vi "PCO_RecorderGetSettings.vi"(0 "phRec":u64, 5 "phCam":u64, 11 "error in (no error)":errorcluster {"code" format="%x"}) -> (2 "wHeight":u16, 3 "dwReqImgCount":u32, 4 "phRec out":u64, 6 "ErrorMessage":i32 format="%x", 8 "dwRecMode":u32, 10 "dwMaxImgCount":u32, 13 "wMetadataLines":u16, 14 "wWidth":u16, 15 "error out":errorcluster {"code" format="%x"})   [LabVIEW 2019, in "Recorder.lvlib"]
doc: "<b>Description:</b>\nThis function retrieves the current recorder settings for a specific camera.\n\n<b>Supported camera type:</b>\nAll cameras"
uses:
  Recorder.lvlib
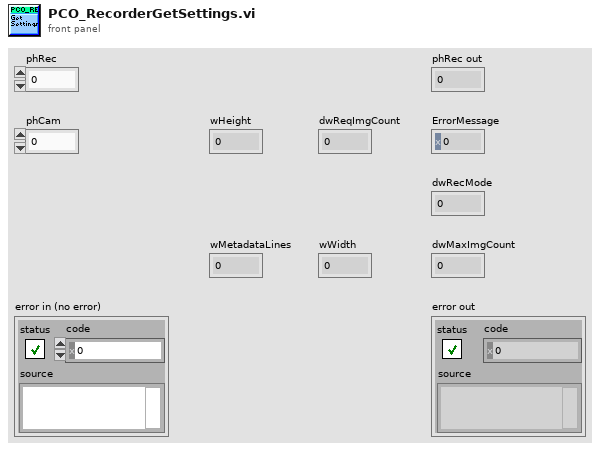
[diagram p1: front panel]
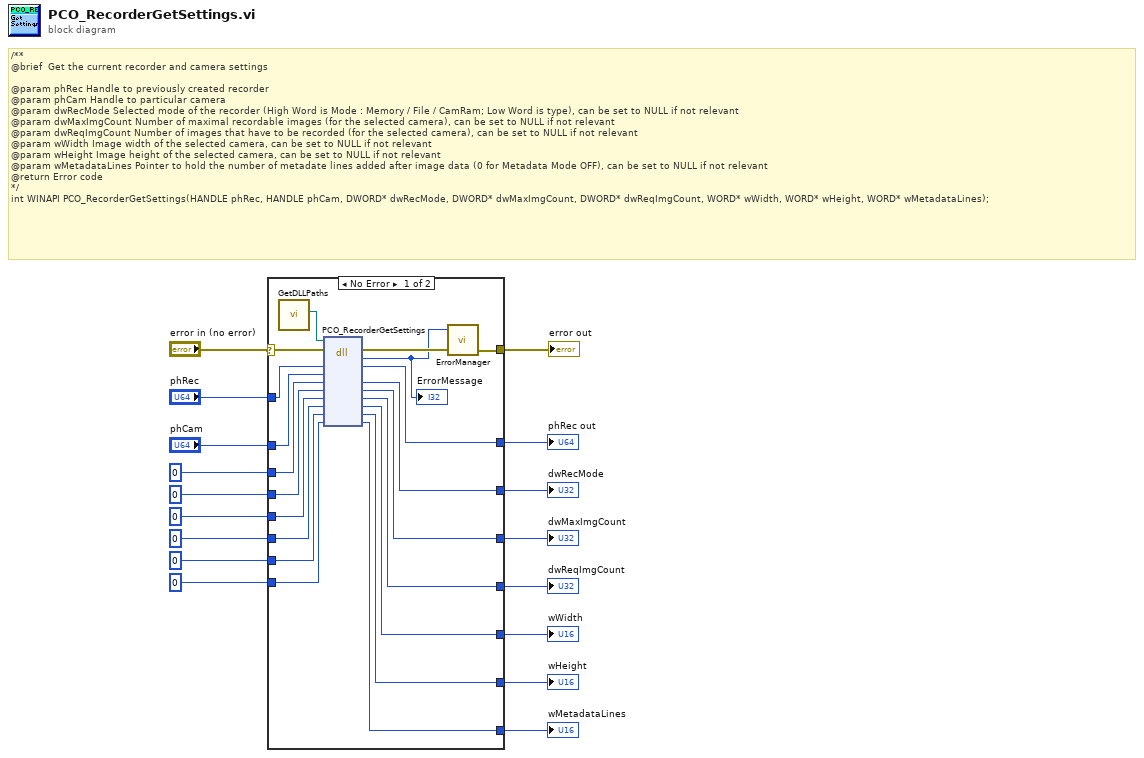
[diagram p0: block diagram]
diagram:
  # "/**\n@brief \tGet the current recorder and camera settings\n\n@param phRec Handle to previously created recorder\n@param phCam Handle to particular camera\n@param dwRecMode Selected mode of the recorder (High Word is Mode : Memory / File / CamRam; Low Word is type), can be set to NULL if not relevant\n@param dwMaxImgCount Number of maximal recordable images (for the selected camera), can be set to NULL if not relevant\n@param dwReqImgCount Number of images that have to be recorded (for the selected camera), can be set to NULL if not relevant\n@param wWidth Image width of the selected camera, can be set to NULL if not relevant\n@param wHeight Image height of the selected camera, can be set to NULL if not relevant\n@param wMetadataLines Pointer to hold the number of metadate lines added after image data (0 for Metadata Mode OFF), can be set to NULL if not relevant\n@return Error code\n*/\nint WINAPI PCO_RecorderGetSettings(HANDLE phRec, HANDLE phCam, DWORD* dwRecMode, DWORD* dwMaxImgCount, DWORD* dwReqImgCount, WORD* wWidth, WORD* wHeight, WORD* wMetadataLines);"
  n1 = case shown="No Error" "error in (no error)" {
    selector: "error in (no error)" -> [w22 w45]
    tunnel: "phRec" -> [w37 w44]
    tunnel: [w36 w44] -> w16
    tunnel: "phCam" -> [w35 _]
    tunnel: u32 0 ("dwRecMode") -> [w34 w43]
    tunnel: [w33 w43] -> w13
    tunnel: u32 0 ("dwMaxImgCount") -> [w32 w42]
    tunnel: [w31 w42] -> w11
    tunnel: u32 0 ("dwReqImgCount") -> [w30 w41]
    tunnel: [w29 w41] -> w9
    tunnel: u16 0 ("wWidth") -> [w28 w40]
    tunnel: [w27 w40] -> w7
    tunnel: u16 0 ("wHeight") -> [w26 w39]
    tunnel: [w25 w39] -> w5
    tunnel: u16 0 ("wMetadataLines") -> [w24 w38]
    tunnel: [w23 w38] -> w3
    tunnel: [w21 w45] -> w2
    frame No Error {
      n2 = call "GetDLLPaths.vi"() -> ("PCO_Recorder_Path"=w18:path)  [unwired: 9 in, 2 out]
      n3 = dll-call lib="?" fn="PCO_RecorderGetSettings"(path in=w18, error in=w22, "phRec"=w37, "phCam"=w35, "dwRecMode"=w34, "dwMaxImgCount"=w32, "dwReqImgCount"=w30, "wWidth"=w28, "wHeight"=w26, "wMetadataLines"=w24) -> (error out=w20:errorcluster, "return type"=w19:i32, "phRec"=w36:u64, "dwRecMode"=w33:u32, "dwMaxImgCount"=w31:u32, "dwReqImgCount"=w29:u32, "wWidth"=w27:u16, "wHeight"=w25:u16, "wMetadataLines"=w23:u16)  [unwired: 2 in, 1 out]
      "ErrorMessage" <- w19
      n4 = call "ErrorManager.vi"("error in (no error)"=w20, "error code"=w19) -> ("error out"=w21:errorcluster)  [unwired: 3 in]
    }
    frame Error {
    }
  }
  "phRec out" <- w16
  "dwRecMode" <- w13
  "dwMaxImgCount" <- w11
  "dwReqImgCount" <- w9
  "wWidth" <- w7
  "wHeight" <- w5
  "wMetadataLines" <- w3
  "error out" <- w2
